vi "Call Abort VI.vi"(8 "error in (no error)":errorcluster, 11 "Assert Message":T1) -> (0 "error out":errorcluster)   [LabVIEW 2018, in "Abort Application Unit Test.lvclass"]
doc: "Wraps up the Abort Application dynamic dispatch call to allow it to be loaded dynamically during unit testing"
uses:
  Abort Application Unit Test.lvclass
  Core/Assert API Components/Message Data.ctl
  Core/Assert API Components/Log Assert Core Components/Failure Actions/Abort Application/Abort Application.lvclass
  Core/Assert API Components/Assert API Components.lvlib
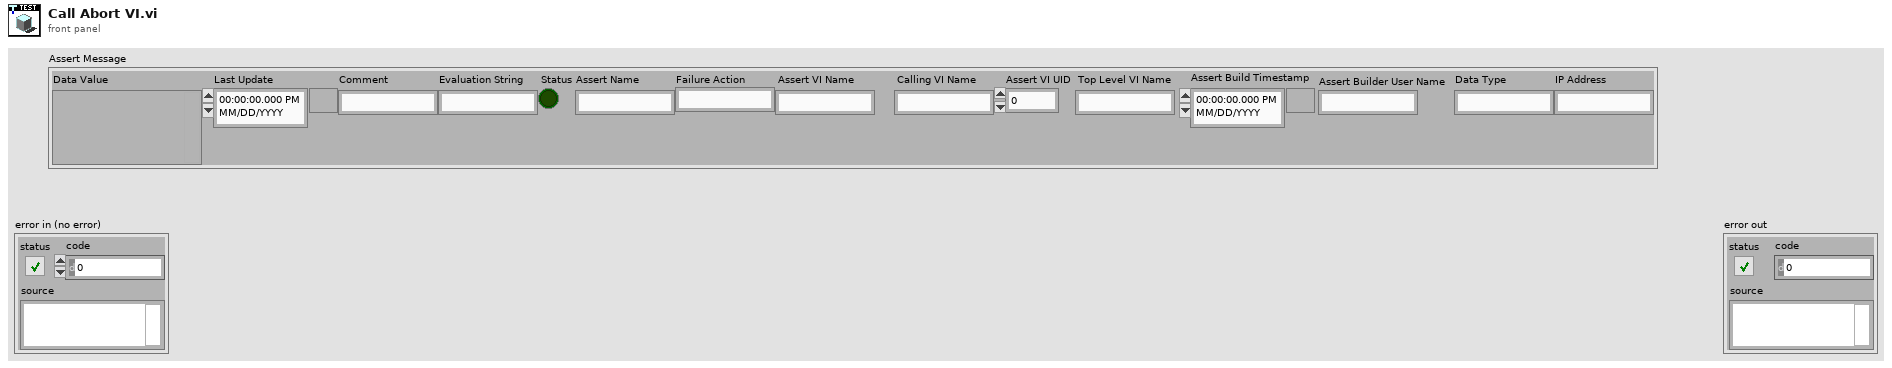
[diagram p1: front panel]
types:
  T1 = typedef "Assert API Components.lvlib/Message Data.ctl" = cluster{"Data Value":variant, "Last Update":timestamp, "Comment":string, "Evaluation String":string, "Status":bool, "Assert Name":string, "Failure Action":string, "Assert VI Name":string, "Calling VI Name":string, "Assert VI UID":i32, "Top Level VI Name":string, "Assert Build Timestamp":timestamp, "Assert Builder User Name":string, "Data Type":string, "IP Address":string}
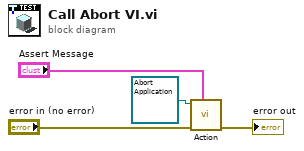
[diagram p0: block diagram]
diagram:
  n1 = call-dynamic "Action.vi"("Assert Message"="Assert Message", "error in (no error)"="error in (no error)", "Abort Application in"=refnum<class "Abort Application.lvclass"> refnum ("Assert API Components.lvlib:Log Assert Core.lvlib:Abort Application.lvclass")) -> ("error out"=→"error out":errorcluster)  [unwired: 8 in]
